vi "SetWaveformBusProperties.vi"(6 "Phase Order":string, 7 "Bus Channel Name":string, 8 "Waveform Channel Order":i32, 9 "Channel Type":string, 10 "Found?":bool, 11 "all channels Wfm":waveform(sgl)[](array[waveform])) -> (3 "all channels Wfm":waveform(sgl)[](array[waveform]))   [LabVIEW 2017, in "McsaVirtualChannel.lvlib"]
uses:
  <vilib>/addons/InsightCM/Devices/Shared/Mcsa/McsaVirtualChannel/McsaVirtualChannel.lvlib
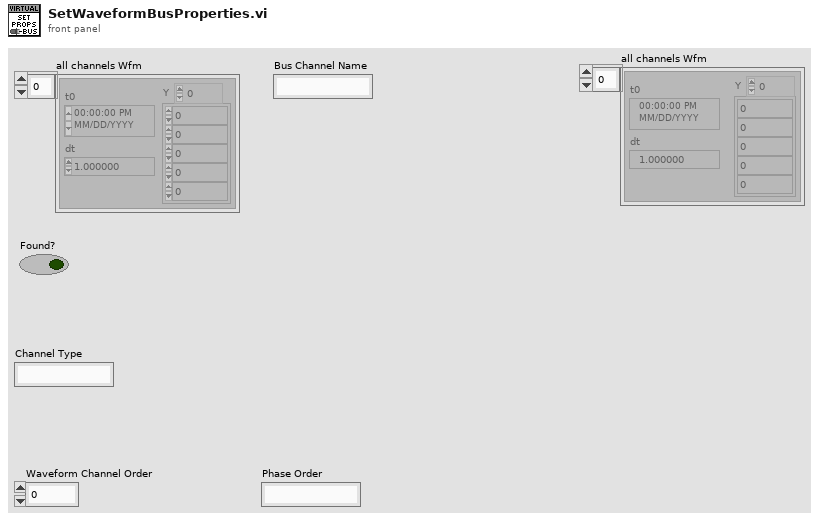
[diagram p1: front panel]
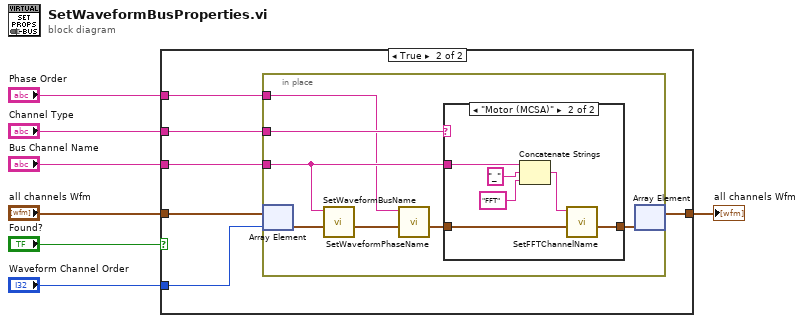
[diagram p0: block diagram]
diagram:
  n1 = case shown="True" "Found?" {
    tunnel: "all channels Wfm" -> [w8 w10]
    tunnel: "Bus Channel Name" -> [_ w12]
    tunnel: "Waveform Channel Order" -> [_ w14]
    tunnel: [w8 w13] -> w3
    tunnel: "Channel Type" -> [_ w11]
    tunnel: "Phase Order" -> [_ w9]
    frame False {
    }
    frame True {
      n2 = in-place {
        in-place-border: w12 -> [w16]
        in-place-border: w11 -> [w17]
        in-place-border: w9 -> [w15]
        n3 = in-place-array #1(w10, w14) -> (w20:waveform(sgl))
        n4 = call <vilib>:"SetWaveformBusName.vi"("Waveform in"=w20, "Name"=w16) -> ("Waveform out"=w21:waveform(sgl))  [unwired: 8 in, 1 out]
        n5 = call <vilib>:"SetWaveformPhaseName.vi"("Waveform in"=w21, "Name"=w15) -> ("Waveform out"=w19:waveform(sgl))  [unwired: 8 in, 1 out]
        n6 = case shown="\"Motor (MCSA)\"" w17 {
          tunnel: w19 -> [w22 w28]
          tunnel: [w22 w27] -> w18
          tunnel: w16 -> [_ w23]
          frame Default {
          }
          frame "Motor (MCSA)" {
            n7 = Concatenate Strings(w23, "_" ("string"), "FFT" ("string")) -> (w24:string)
            n8 = call <vilib>:"SetFFTChannelName.vi"("Waveform in"=w28, "Name"=w24) -> ("Waveform out"=w27:waveform(sgl))  [unwired: 8 in, 1 out]
          }
        }
        n9 = in-place-array #1(w18) -> (w13:waveform(sgl)[])  [unwired: 1 out]
      }
    }
  }
  "all channels Wfm" <- w3
